vi "ParseArguments.vi"(8 "error in (no error)":errorcluster, 9 "Inputs":string[](array[string]), 11 "MassCompile in":refnum<class "MassCompile.lvclass">) -> (0 "error out":errorcluster, 3 "MassCompile out":refnum<class "MassCompile.lvclass">)   [LabVIEW 2014, in "MassCompile.lvclass"]
uses:
  MassCompile.lvclass
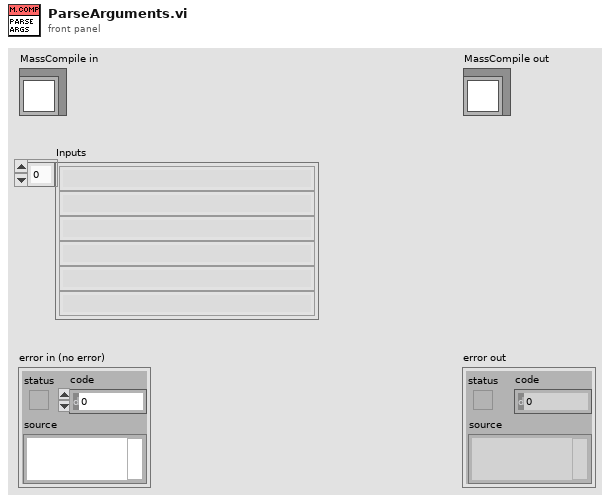
[diagram p1: front panel]
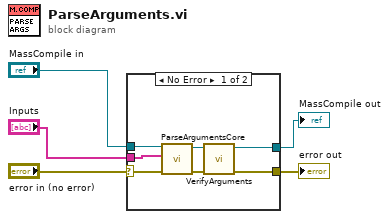
[diagram p0: block diagram]
diagram:
  n1 = case shown="No Error" "error in (no error)" {
    selector: "error in (no error)" -> [w7 w13]
    tunnel: "MassCompile in" -> [w12 w14]
    tunnel: "Inputs" -> [w11 _]
    tunnel: [w8 w14] -> w3
    tunnel: [w6 w13] -> w1
    frame No Error {
      n2 = call "ParseArgumentsCore.vi"("error in (no error)"=w7, "Inputs"=w11, "MassCompile in"=w12) -> ("error out"=w9:errorcluster, "MassCompile out"=w10:refnum<class "MassCompile.lvclass">)  [unwired: 7 in]
      n3 = call "VerifyArguments.vi"("error in (no error)"=w9, "MassCompile in"=w10) -> ("error out"=w6:errorcluster, "MassCompile out"=w8:refnum<class "MassCompile.lvclass">)  [unwired: 8 in]
    }
    frame Error {
    }
  }
  "error out" <- w1
  "MassCompile out" <- w3
